vi "example_01_build_graph.vi"() -> ()   [LabVIEW 2015, in "lv-graph.lvlib"]
doc: "This is an example meant to showcase different graphs being built from the same/similar data, it shows a single plot, a multi-plot and a vertical strip chart graph. The data rate can be configured and the data grows infinitely. It can be configured for \"real-time\" data by setting the boolean from Random to Real-time. Note that the multi-plot will fail when realtime is used (because i'm lazy), look deeper to find out why."
uses:
  advanced/build_graph-single_axis.vi
  advanced/build_graph-vertical.vi
  advanced/build_graph-multiple_axis.vi
  lv-graph.lvlib
panel:
  out "multiple_plot":T1(graph)
  out "vertical_strip":T2(graph)
  in  "realtime":bool
  in  "data_rate_ms":u32=10
  in  "stop":bool
  out "single_plot":T1(graph)
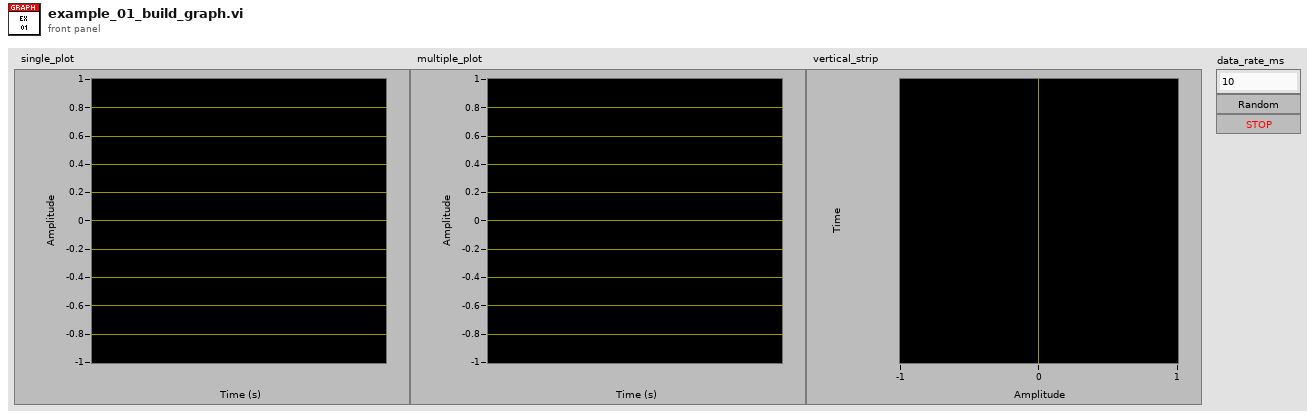
[diagram p1: front panel]
types:
  T1 = cluster{"Time [] out":dbl[], "Data[][] out":dbl[]}[]
  T2 = cluster{cluster{"Timestamp":dbl, "Timestamp":dbl}[]}[]
  T3 = cluster{"x_scale_maximum":dbl, "x_scale_minimum":dbl, "y_scale_maximum":dbl, "y_scale_minimum":dbl}
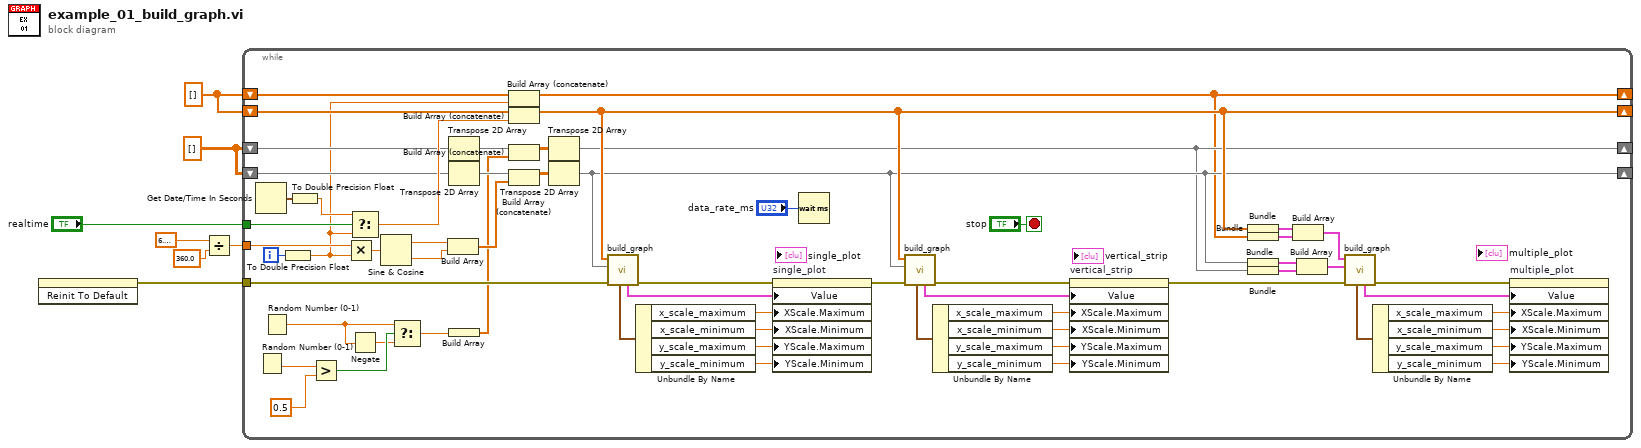
[diagram p0: block diagram]
diagram:
  w1 = dbl[][] []
  w2 = dbl[] []
  n1 = invoke on="stop" class="Bool" method="Reinit To Default"() -> (error out=w3:errorcluster)  [unwired: 3 in, 2 out]
  n2 = Divide(x=6.283185307179586, y=360.0) -> (x/y=w4:dbl)
  n3 = while {
    tunnel: w3 -> [w51]
    shift-right: [w25] -> _
    shift-left: w2 -> [w55]
    shift-right: [w24] -> _
    shift-left: w1 -> [w52]
    tunnel: "realtime" -> [w58]
    tunnel: w4 -> [w57]
    shift-right: [w15] -> _
    shift-left: w2 -> [w22]
    shift-right: [w16] -> _
    shift-left: w1 -> [w18]
    i -> [w56]
    stop <- "stop" stop-if-true
    n4 = Get Date/Time In Seconds() -> (seconds since 1Jan1904=w59:timestamp)
    n5 = Random Number (0-1)() -> (number: 0 to 1=w13:dbl)
    n6 = Random Number (0-1)() -> (number: 0 to 1=w10:dbl)
    n7 = To Double Precision Float(number=w56) -> (double precision float=w14:dbl)
    n8 = To Double Precision Float(number=w59) -> (double precision float=w21:dbl)
    n9 = Greater?(x=w13, y=0.5) -> (0:w11:bool)
    n10 = Multiply(x=w57, y=w14) -> (x*y=w60:dbl)
    n11 = Select(t=w21, s=w58, f=w14) -> (s? t:f=w54:dbl)
    n12 = Negate(x=w10) -> (-x=w8:dbl)
    n13 = Sine & Cosine(0:w60) -> (1:w61:dbl, 2:w62:dbl)
    n14 = Select(t=w10, s=w11, f=w8) -> (s? t:f=w9:dbl)
    n15 = Build Array(w61, w62) -> (w53:dbl[])
    n16 = Transpose 2D Array(2D array=w18) -> (transposed array=w20:dbl[][])
    n17 = Transpose 2D Array(2D array=w52) -> (transposed array=w49:dbl[][])
    n18 = Build Array(w9) -> (w17:dbl[])
    n19 = Build Array (concatenate)(w22, w14) -> (w15:dbl[])
    n20 = Build Array (concatenate)(w55, w54) -> (w25:dbl[])
    n21 = Build Array (concatenate)(w20, w17) -> (w19:dbl[][])
    n22 = Build Array (concatenate)(w49, w53) -> (w50:dbl[][])
    n23 = Transpose 2D Array(2D array=w19) -> (transposed array=w16:dbl[][])
    n24 = Transpose 2D Array(2D array=w50) -> (transposed array=w24:dbl[][])
    n25 = call-poly "build_graph.vi"("error in (no error)"=w51, "y_axis"=w24, "x_axis"=w25) -> ("error out"=w68:errorcluster, "graph_data"=w41:cluster{dbl[], dbl[]}[], "scale_ranges"=w42:T3)  [unwired: 6 in]
    n26 = Unbundle By Name(w42) -> ("x_scale_maximum"=w66:dbl, "x_scale_minimum"=w67:dbl, "y_scale_maximum"=w65:dbl, "y_scale_minimum"=w64:dbl)
    n27 = property on="single_plot" class="XYGraph (strict)"(error in=w68, "Value"=w41, "XScale.Maximum"=w66, "XScale.Minimum"=w67, "YScale.Maximum"=w65, "YScale.Minimum"=w64) -> (error out=w46:errorcluster)  [unwired: 1 in, 1 out]
    n28 = Wait (ms)(milliseconds to wait="data_rate_ms") -> ()  [unwired: 1 out]
    n29 = call-poly "build_graph.vi"("error in (no error)"=w46, "y_axis"=w24, "x_axis"=w25) -> ("error out"=w45:errorcluster, "graph_data"=w39:T2, "scale_ranges"=w40:T3)  [unwired: 6 in]
    n30 = Unbundle By Name(w40) -> ("x_scale_maximum"=w48:dbl, "x_scale_minimum"=w47:dbl, "y_scale_maximum"=w44:dbl, "y_scale_minimum"=w43:dbl)
    n31 = property on="vertical_strip" class="XYGraph (strict)"(error in=w45, "Value"=w39, "XScale.Maximum"=w48, "XScale.Minimum"=w47, "YScale.Maximum"=w44, "YScale.Minimum"=w43) -> (error out=w33:errorcluster)  [unwired: 1 in, 1 out]
    n32 = Bundle(w25) -> (w26:cluster{dbl[]})  [unwired: 1 in]
    n33 = Bundle(w15) -> (w27:cluster{dbl[]})  [unwired: 1 in]
    n34 = Bundle(w24) -> (w29:cluster{dbl[][]})  [unwired: 1 in]
    n35 = Bundle(w16) -> (w28:cluster{dbl[][]})  [unwired: 1 in]
    n36 = Build Array(w26, w27) -> (w31:cluster{dbl[]}[])
    n37 = Build Array(w29, w28) -> (w30:cluster{dbl[][]}[])
    n38 = call-poly "build_graph.vi"("error in (no error)"=w33, "y_axis"=w30, "x_axis"=w31) -> ("error out"=w37:errorcluster, "graph_data"=w32:cluster{dbl[], dbl[]}[], "scale_range"=w34:T3)  [unwired: 6 in]
    n39 = Unbundle By Name(w34) -> ("x_scale_maximum"=w35:dbl, "x_scale_minimum"=w36:dbl, "y_scale_maximum"=w38:dbl, "y_scale_minimum"=w23:dbl)
    n40 = property on="multiple_plot" class="XYGraph (strict)"(error in=w37, "Value"=w32, "XScale.Maximum"=w35, "XScale.Minimum"=w36, "YScale.Maximum"=w38, "YScale.Minimum"=w23) -> ()  [unwired: 1 in, 2 out]
  }
